vi "FW-EnQueueMultiOrderss.vi"(7 "CMDs":cluster{"cmd":T1, "Param":variant}[](array[cluster]), 8 "ErrorIn":errorcluster, 11 "QueueIn":refnum<queue>) -> (0 "ErrorOut":errorcluster, 3 "QueueOut":refnum<queue>)   [LabVIEW 2020]
doc: "Enqueue Multi Elements\n- Enqueue all elements in arrary to queue.\n\nNotes:\n- N/A"
uses:
  Cmd.ctl
panel:
  # "Inputs"
  # "Outputs"
  # ":: Modularized Parallism Templete ::\n- EnQueue MultiElements -\nby: Techie <HighTechYoung@yahoo.com>\nCopyright (C) 2010, Vision Technologies All Rights Reserved"
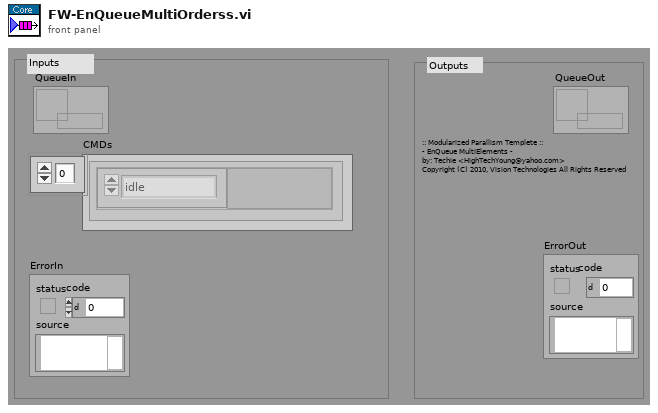
[diagram p1: front panel]
types:
  T1 = typedef "Cmd.ctl" = enum16{"idle", "---------- APP ---------", "APP::Init", "APP::Exit", "-------- ERROR --------", "ERR::Handler", "------ TEST PLAN ------", "TEST::Prep", "TEST::Start", "TEST::Run", "TEST::Pause", "TEST::Exit", "---- MACHINE VISION----", "MV::Init", "MV::Prep", "MV::SetROI", "MV::Cord", "MV::Check", "MV::Clean", "--------- USER ----------", "USER::Case1", "USER::Case2"}
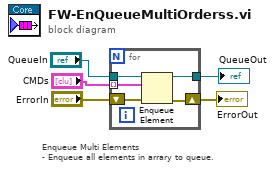
[diagram p0: block diagram]
diagram:
  # "Enqueue Multi Elements\n- Enqueue all elements in arrary to queue."
  n1 = for {
    shift-right: [w9] -> w4
    shift-left: "ErrorIn" -> [w10]
    tunnel: "QueueIn" -> [w8]
    tunnel: "CMDs" -> [w7] mode=indexing
    tunnel: [w6] -> w1
    n2 = Enqueue Element(queue=w8, element=w7, error in (no error)=w10) -> (queue out=w6:refnum<queue>, error out=w9:errorcluster)  [unwired: 2 out]
  }
  "ErrorOut" <- w4
  "QueueOut" <- w1
